vi "Target_9.vi"   [LabVIEW 2020]
uses:
  <vilib>/Platform/TimedLoop/XDataNode/timing_clust.ctl
  <vilib>/Platform/TimedLoop/XDataNode/nitl_modes.ctl
  <vilib>/Platform/TimedLoop/XDataNode/wakeup.ctl
  <vilib>/platform/TimedLoop/XDataNode/XDataNode.xnode
  <vilib>/Platform/TimedLoop/XDataNode/XDNodeRunTimeDep.lvlib
types:
  T1 = typedef "XDNodeRunTimeDep.lvlib/timing_clust.ctl" = cluster{"Expected End [f-1]":u64, "Actual End [f-1]":u64, "Finished Late? [f-1]":bool, "Expected End [i-1]":u64, "Actual End [i-1]":u64, "Finished Late? [i-1]":bool, "Expected Start [i]":u64, "Actual Start [i]":u64, "Expected Start [f]":u64, "Actual Start [f]":u64, "Source Name":string, "Structure Name":string, "Period":i64, "Deadline":i64, "Offset":i64, "Start":i64, "Priority":i32, "Timeout":i32, "Mode":T2, "Wakeup Reason":T3, "Error":errorcluster, "Source Type":string, "Secondary Source Type":string, "Global End Time":u64, "Global Start Time":u64, "Frame Duration":u64, "Iteration Duration":u64, "Assigned CPU":i32, "I/O Scan Engine Mode":u32}
  T2 = typedef "XDNodeRunTimeDep.lvlib/nitl_modes.ctl" = enum32{"No Change", "Process missed periods, maintain original phase", "Discard missed periods, maintain original phase", "Process missed periods, ignore original phase", "Discard missed periods, ignore original phase"}
  T3 = typedef "XDNodeRunTimeDep.lvlib/wakeup.ctl" = enum32{"Normal", "Aborted", "Asynchronous wakeup", "Timing source error", "Timed loop error", "Timeout"}
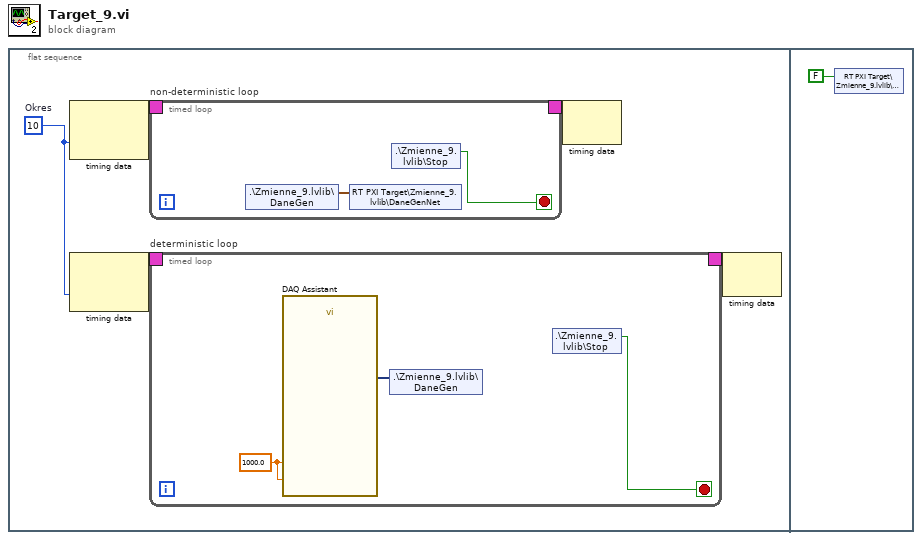
[diagram p0: block diagram]
diagram:
  n1 = flat-sequence {
    frame #0 {
      w1 = i64 10  # Okres
      n2 = node-c288 ("Input Node")(w1) -> (w3:T1)  [unwired: 1 in]
      n3 = node-c288 ("Input Node")(w1) -> (w5:T1)  [unwired: 1 in]
      n4 = timed-loop "non-deterministic loop" {
        timing: w3 -> [_]
        timing-out: [_] -> w2
        stop <- w7 stop-if-true
        n5 = shared-variable ".\\Zmienne_9.lvlib\\DaneGen"() -> (w6:waveform(dbl))  [unwired: 1 in, 1 out]
        n6 = shared-variable "RT PXI Target\\Zmienne_9.lvlib\\DaneGenNet"(w6) -> ()  [unwired: 1 in, 1 out]
        n7 = shared-variable ".\\Zmienne_9.lvlib\\Stop"() -> (w7:bool)  [unwired: 1 in, 1 out]
      }
      n8 = timed-loop "deterministic loop" {
        timing: w5 -> [_]
        timing-out: [_] -> w4
        stop <- w16 stop-if-true
        w15 = 1000.0 ("rate")
        n9 = call "DAQ Assistant"("rate"=w15, "number of samples"=w15) -> ("data"=w14:dynamicdata)  [unwired: 15 in, 2 out]
        n10 = shared-variable ".\\Zmienne_9.lvlib\\DaneGen"(w14) -> ()  [unwired: 1 in, 1 out]
        n11 = shared-variable ".\\Zmienne_9.lvlib\\Stop"() -> (w16:bool)  [unwired: 1 in, 1 out]
      }
      n12 = node-c288 ("Output Node")(w2) -> ()  [unwired: 1 out]
      n13 = node-c288 ("Output Node")(w4) -> ()  [unwired: 1 out]
    }
    frame #1 {
      n14 = shared-variable "RT PXI Target\\Zmienne_9.lvlib\\Stop"(FALSE ("Stop")) -> ()  [unwired: 1 in, 1 out]
    }
  }
